vi "Finish_LDA.vi"() -> (1 "LDA Binary output":u16[][](array[numeric])=[[142, 132, 123, 114, 103, 93, 84, 74, 65, 56, 49, 42, 35, 30, 27, 24, 23, 22, 24, 26, 30, 35, 41, 48, 56, 65, 73, 82, 93, 102, 112, 122, 132, 141, 149, 156, 164, 169, 173, 177, 180, 181, 181, 179, 176, 171, 167, 160, 153, 145, 137, 128, 118, 108, 98, 88, 79, 69, 61, 52, 45, 38, 33, 28, 25, 23, 22, 23, 25, 29, 32, 39, 45, 52, 60, 69, 78, 88, 97, 108, 118, 127, 136, 145, 153, 160, 166, 171, 176, 179, 180, 181, 180, 178, 174, 169, 164, 157, 149, 141]], 4 "Repeat Block":bool)   [LabVIEW 2010]
doc: "The Getting Started Analog Input VI illustrates the basic concepts involved in acquiring analog input data from any data acquisition hardware.\n\nThis VI is explained in detail in the Getting Started with Analog Input section of chapter 1 of the Data Acquisition VI Reference Manual. If you are using SCXI, you should read the Getting Started with SCXI section of chapter 1 first.\n\nAfter you have installed and configured your data acquisition hardware as described in the Installation and Configuration section of chapter 1, you can run this VI to verify your hardware configuration. \n\nYou can pop-up on any front panel object for a description.\n\nIf you are using AMUX-64T boards or SCXI hardware, look at the channels control description for instructions on how to address those external channels; otherwise, you can run the VI with default inputs.\n\nOpen the diagram window to see the data acquisition VI usage."
uses:
  Globals/LDA_meas_global_1.vi
  Globals/Meas_global.vi
  Globals/LDA_meas_global_2.vi
panel:
  out "error out":errorcluster
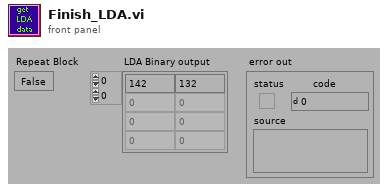
[diagram p1: front panel]
types:
  T1 = typedef "BSA_info_Cluster.ctl" = cluster{"GPIB Address":string, "No of Check Bytes":i32, "Extra Info":string, "COLOUR":u32, "Wavelength (nm)":dbl}
  T2 = cluster{"Burst criterion":enum16{"Envelope", "Pedestal", "Env and ped"}, "Oversize reject level":enum16{"1 (disabled)", "2", "3", "4", "5", "6", "7", "8", "9"}, "Pedestal attenuation":enum16{"0", "6", "12", "18"}, "Record length":enum16{"8", "16", "32", "64"}, "Quality factor":i16}
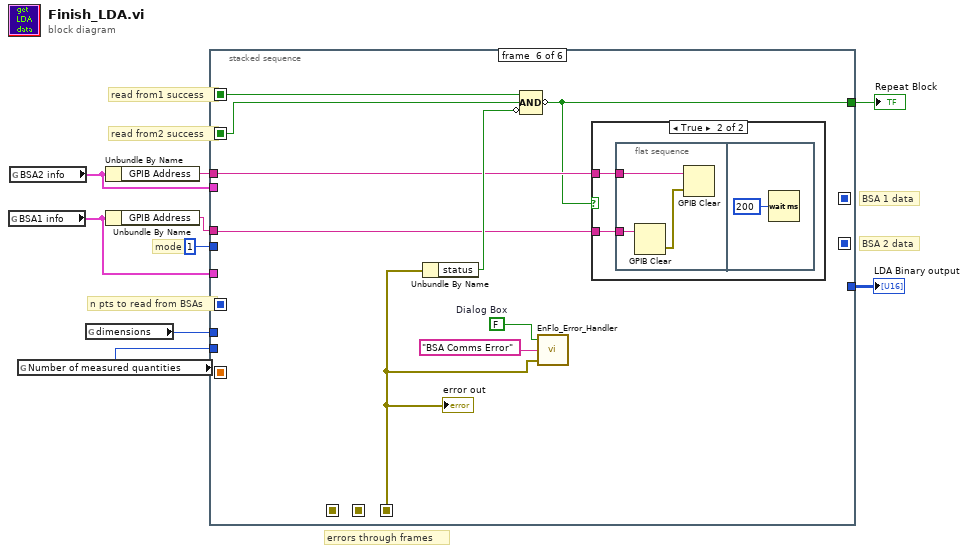
[diagram p0: block diagram]
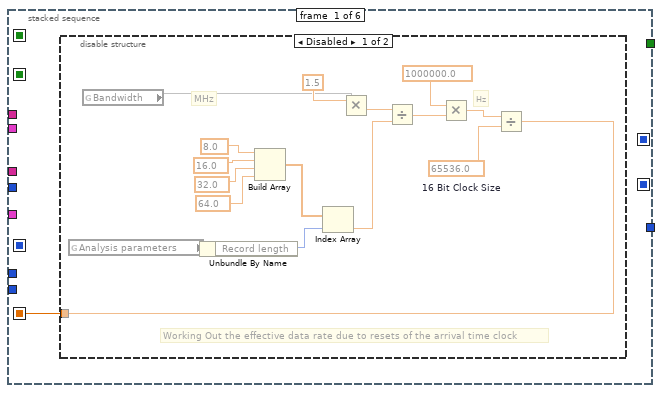
[diagram p2: hidden frame]
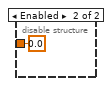
[diagram p3: hidden frame]
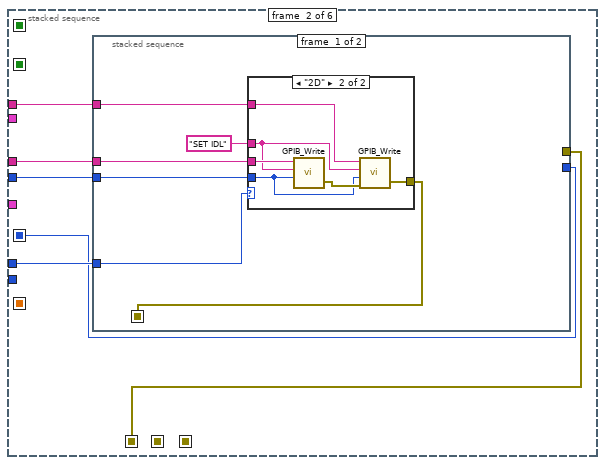
[diagram p4: hidden frame]
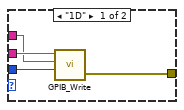
[diagram p5: hidden frame]
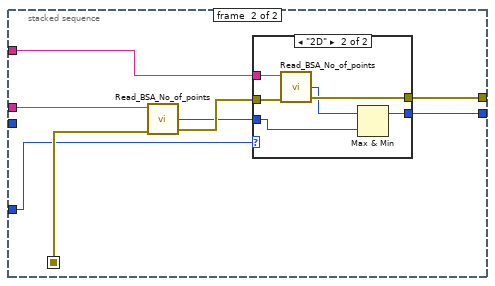
[diagram p6: hidden frame]
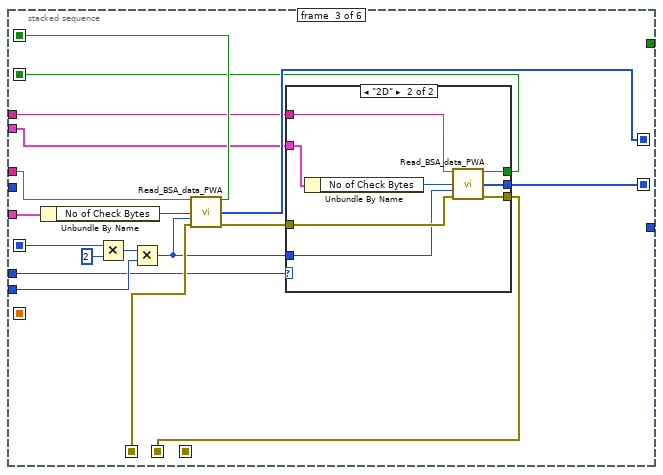
[diagram p8: hidden frame]
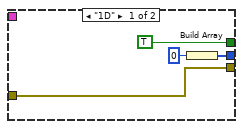
[diagram p9: hidden frame]
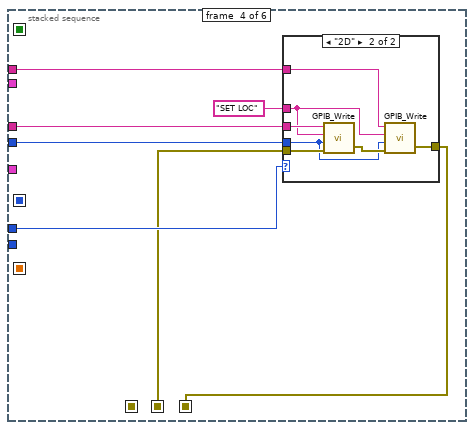
[diagram p10: hidden frame]
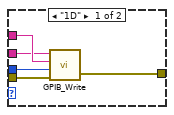
[diagram p11: hidden frame]
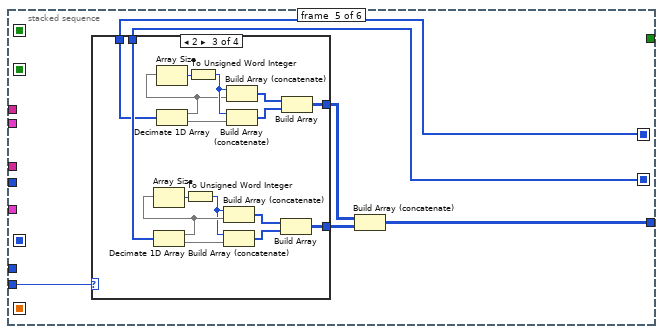
[diagram p12: hidden frame]
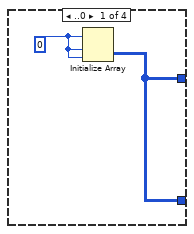
[diagram p13: hidden frame]
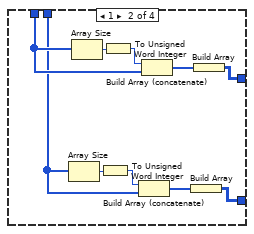
[diagram p14: hidden frame]
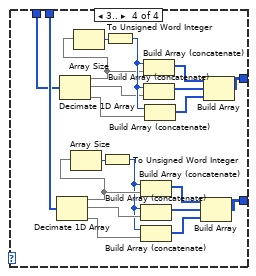
[diagram p15: hidden frame]
diagram:
  # "errors through frames"
  # "BSA 2 data"
  # "BSA 1 data"
  # "read from2 success"
  # "read from1 success"
  # "mode"
  # "n pts to read from BSAs"
  n1 = global read "LDA_meas_global_1.vi" "BSA1 info"() -> (w1:T1)
  n2 = global read "LDA_meas_global_2.vi" "BSA2 info"() -> (w2:T1)
  n3 = global read "LDA_meas_global_1.vi" "Number of measured quantities"() -> (w8:i32)
  n4 = global read "Meas_global.vi" "dimensions"() -> (w6:enum16{"1D", "2D"})
  n5 = Unbundle By Name(w2) -> ("GPIB Address"=w3:string)
  n6 = Unbundle By Name(w1) -> ("GPIB Address"=w7:string)
  n7 = stacked-sequence {
    seq-local: [_ _ w78 _ _ _] -> [_ _ _ _ w119 _]
    seq-local: [_ _ w70 _ _ _] -> [_ _ _ _ w118 _]
    seq-local: [_ _ w82 _ _ _] -> [_ _ _ _ _ w177]
    seq-local: [_ _ w73 _ _ _] -> [_ _ _ _ _ w176]
    seq-local: [_ w28 _ _ _ _] -> [_ _ w75 _ _ _]
    seq-local: [_ _ _ w96 _ _] -> [_ _ _ _ _ w172]
    seq-local: [_ w29 _ _ _ _] -> [_ _ w77 _ _ _]
    seq-local: [w10 _ _ _ _ _] -> [_ _ _ _ _ _]
    seq-local: [_ _ w67 _ _ _] -> [_ _ _ w97 _ _]
    tunnel: w8 -> [_ _ w83 _ w120 _]
    tunnel: i16 1 -> [_ w32 _ w102 _ _]
    tunnel: w7 -> [_ w33 w76 w100 _ w171]
    tunnel: w6 -> [_ w31 w66 w99 _ _]
    tunnel: [_ _ _ _ w115 _] -> w5
    tunnel: [_ _ _ _ _ w169] -> w4
    tunnel: w3 -> [_ w30 w72 w98 _ w170]
    tunnel: w1 -> [_ _ w74 _ _ _]
    tunnel: w2 -> [_ _ w71 _ _ _]
    frame #0 {
      n8 = disable-structure shown="Disabled" {
        disable-tunnel: [w11 0.0] -> w10
        frame Disabled {
          w20 = 65536.0  # 16 Bit Clock Size
          # "Hz"
          # "MHz"
          # "Working Out the effective data rate due to resets of the arrival time clock"
          n9 = global read "LDA_meas_global_1.vi" "Analysis parameters"() -> (w19:T2)
          n10 = global read "LDA_meas_global_1.vi" "Bandwidth"() -> (w25)
          n11 = Unbundle By Name(w19) -> ("Record length"=w13:enum16{"8", "16", "32", "64"})
          n12 = Build Array(8.0, 16.0, 32.0, 64.0) -> (w14:dbl[])
          n13 = Index Array(array=w14, index=w13) -> (element=w12:dbl)
          n14 = Multiply(x=1.5, y=w25) -> (x*y=w24:dbl)
          n15 = Divide(x=w24, y=w12) -> (x/y=w23:dbl)
          n16 = Multiply(x=1000000.0, y=w23) -> (x*y=w21:dbl)
          n17 = Divide(x=w21, y=w20) -> (x/y=w11:dbl)
        }
        frame Enabled {
        }
      }
    }
    frame #1 {
      n18 = stacked-sequence {
        seq-local: [w37 _] -> [_ w56]
        tunnel: w33 -> [w39 w57]
        tunnel: w32 -> [w38 _]
        tunnel: w31 -> [w36 w51]
        tunnel: w30 -> [w34 w55]
        tunnel: [_ w52] -> w29
        tunnel: [_ w50] -> w28
        frame #0 {
          n19 = case shown="\"2D\"" w36 {
            tunnel: w39 -> [w43 w49]
            tunnel: w38 -> [w42 w44]
            tunnel: [w41 w47] -> w37
            tunnel: "SET IDL" -> [w40 w45]
            tunnel: w34 -> [_ w46]
            frame "1D" {
              n20 = call "GPIB_Write.vi"("address string"=w43, "data In"=w40, "mode (0)"=w42) -> ("error out"=w41:errorcluster)  [unwired: 2 in, 1 out]
            }
            frame "2D" {
              n21 = call "GPIB_Write.vi"("address string"=w49, "data In"=w45, "mode (0)"=w44) -> ("error out"=w48:errorcluster)  [unwired: 2 in, 1 out]
              n22 = call "GPIB_Write.vi"("address string"=w46, "data In"=w45, "mode (0)"=w44, "error in"=w48) -> ("error out"=w47:errorcluster)  [unwired: 1 in, 1 out]
            }
          }
        }
        frame #1 {
          n23 = call "Read_BSA_No_of_points.vi"("error in (no error)"=w56, "GPIB Address"=w57) -> ("error out"=w54:errorcluster, "No of samples"=w53:i32)  [unwired: 3 out]
          n24 = case shown="\"2D\"" w51 {
            tunnel: w54 -> [w59 w65]
            tunnel: w55 -> [_ w64]
            tunnel: [w59 w63] -> w50
            tunnel: w53 -> [w58 w61]
            tunnel: [w58 w60] -> w52
            frame "1D" {
            }
            frame "2D" {
              n25 = call "Read_BSA_No_of_points.vi"("error in (no error)"=w65, "GPIB Address"=w64) -> ("error out"=w63:errorcluster, "No of samples"=w62:i32)  [unwired: 3 out]
              n26 = Max & Min(x=w62, y=w61) -> (max(x,y)=w60:i32)  [unwired: 1 out]
            }
          }
        }
      }
    }
    frame #2 {
      n27 = Unbundle By Name(w74) -> ("No of Check Bytes"=w79:i32)
      n28 = Multiply(x=w77, y=2) -> (x*y=w80:i32)
      n29 = Multiply(x=w80, y=w83) -> (x*y=w68:i32)
      n30 = call "Read_BSA_data_PWA.vi"("GPIB Address"=w76, "No of Check Bytes"=w79, "Bytes per block"=w68, "error in (no error)"=w75) -> ("transmission okay"=w82:bool, "array of velocity data"=w78:u16[], "error out"=w69:errorcluster)  [unwired: 9 out]
      n31 = case shown="\"2D\"" w66 {
        tunnel: [w86 w95] -> w70
        tunnel: [TRUE ("transmission okay") w93] -> w73
        tunnel: [w84 w89] -> w67
        tunnel: w71 -> [_ w92]
        tunnel: w72 -> [_ w91]
        tunnel: w69 -> [w84 w90]
        tunnel: w68 -> [_ w88]
        frame "1D" {
          n32 = Build Array(u16 0) -> (w86:u16[])
        }
        frame "2D" {
          n33 = Unbundle By Name(w92) -> ("No of Check Bytes"=w94:i32)
          n34 = call "Read_BSA_data_PWA.vi"("GPIB Address"=w91, "No of Check Bytes"=w94, "Bytes per block"=w88, "error in (no error)"=w90) -> ("transmission okay"=w93:bool, "array of velocity data"=w95:u16[], "error out"=w89:errorcluster)  [unwired: 9 out]
        }
      }
    }
    frame #3 {
      n35 = case shown="\"2D\"" w99 {
        tunnel: w102 -> [w107 w110]
        tunnel: "SET LOC" -> [w106 w109]
        tunnel: w100 -> [w105 w114]
        tunnel: w97 -> [w104 w113]
        tunnel: [w103 w111] -> w96
        tunnel: w98 -> [_ w108]
        frame "1D" {
          n36 = call "GPIB_Write.vi"("address string"=w105, "data In"=w106, "mode (0)"=w107, "error in"=w104) -> ("error out"=w103:errorcluster)  [unwired: 1 in, 1 out]
        }
        frame "2D" {
          n37 = call "GPIB_Write.vi"("address string"=w114, "data In"=w109, "mode (0)"=w110, "error in"=w113) -> ("error out"=w112:errorcluster)  [unwired: 1 in, 1 out]
          n38 = call "GPIB_Write.vi"("address string"=w108, "data In"=w109, "mode (0)"=w110, "error in"=w112) -> ("error out"=w111:errorcluster)  [unwired: 1 in, 1 out]
        }
      }
    }
    frame #4 {
      n39 = case shown="2" w120 {
        tunnel: w119 -> [_ w124 w133 w149]
        tunnel: w118 -> [_ w123 w148 w168]
        tunnel: [w121 w132 w147 w167] -> w117
        tunnel: [w121 w131 w146 w166] -> w116
        frame ..0 {
          w122 = u16 0
          n40 = Initialize Array(w122, w122, w122) -> (w121:u16[][])
        }
        frame 1 {
          n41 = Array Size(array=w123) -> (size(s)=w130:i32)
          n42 = Array Size(array=w124) -> (size(s)=w125:i32)
          n43 = To Unsigned Word Integer(number=w130) -> (unsigned 16bit integer=w129:u16)
          n44 = To Unsigned Word Integer(number=w125) -> (unsigned 16bit integer=w126:u16)
          n45 = Build Array (concatenate)(w129, w123) -> (w128:u16[])
          n46 = Build Array (concatenate)(w126, w124) -> (w127:u16[])
          n47 = Build Array(w128) -> (w131:u16[][])
          n48 = Build Array(w127) -> (w132:u16[][])
        }
        frame 2 {
          n49 = Decimate 1D Array(w148) -> (w145:u16[], w143:u16[])
          n50 = Array Size(array=w145) -> (size(s)=w144:i32)
          n51 = Decimate 1D Array(w133) -> (w134:u16[], w136:u16[])
          n52 = Array Size(array=w134) -> (size(s)=w135:i32)
          n53 = To Unsigned Word Integer(number=w144) -> (unsigned 16bit integer=w142:u16)
          n54 = To Unsigned Word Integer(number=w135) -> (unsigned 16bit integer=w137:u16)
          n55 = Build Array (concatenate)(w142, w145) -> (w141:u16[])
          n56 = Build Array (concatenate)(w142, w143) -> (w140:u16[])
          n57 = Build Array (concatenate)(w137, w134) -> (w138:u16[])
          n58 = Build Array (concatenate)(w137, w136) -> (w139:u16[])
          n59 = Build Array(w141, w140) -> (w146:u16[][])
          n60 = Build Array(w138, w139) -> (w147:u16[][])
        }
        frame 3.. {
          n61 = Decimate 1D Array(w168) -> (w165:u16[], w163:u16[], w162:u16[])
          n62 = Decimate 1D Array(w149) -> (w150:u16[], w152:u16[], w153:u16[])
          n63 = Array Size(array=w165) -> (size(s)=w164:i32)
          n64 = Array Size(array=w150) -> (size(s)=w151:i32)
          n65 = To Unsigned Word Integer(number=w164) -> (unsigned 16bit integer=w161:u16)
          n66 = To Unsigned Word Integer(number=w151) -> (unsigned 16bit integer=w154:u16)
          n67 = Build Array (concatenate)(w161, w165) -> (w160:u16[])
          n68 = Build Array (concatenate)(w161, w163) -> (w159:u16[])
          n69 = Build Array (concatenate)(w161, w162) -> (w158:u16[])
          n70 = Build Array (concatenate)(w154, w150) -> (w155:u16[])
          n71 = Build Array (concatenate)(w154, w152) -> (w156:u16[])
          n72 = Build Array (concatenate)(w154, w153) -> (w157:u16[])
          n73 = Build Array(w160, w159, w158) -> (w166:u16[][])
          n74 = Build Array(w155, w156, w157) -> (w167:u16[][])
        }
      }
      n75 = Build Array (concatenate)(w117, w116) -> (w115:u16[][])
    }
    frame #5 {
      w175 = FALSE  # Dialog Box
      n76 = Unbundle By Name(w172) -> ("status"=w173:bool)
      n77 = Compound Arithmetic op=AND(w177, w176, invert w173) -> (invert w169:bool)
      n78 = call "EnFlo_Error_Handler.vi"("error in (no error)"=w172, "Error Type"="BSA Comms Error", "Dialog Box (T)"=w175) -> ()  [unwired: 3 out]
      n79 = case shown="True" w169 {
        tunnel: w171 -> [_ w179]
        tunnel: w170 -> [_ w178]
        frame False {
        }
        frame True {
          n80 = flat-sequence {
            tunnel: w179 -> [w182]
            tunnel: w178 -> [w181]
            frame #0 {
              n81 = GPIB Clear(3:w182) -> (0:w180:errorcluster)  [unwired: 1 in, 1 out]
              n82 = GPIB Clear(2:w180, 3:w181) -> ()  [unwired: 2 out]
            }
            frame #1 {
              n83 = Wait (ms)(milliseconds to wait=u32 200) -> ()  [unwired: 1 out]
            }
          }
        }
      }
      "error out" <- w172
    }
  }
  "LDA Binary output" <- w5
  "Repeat Block" <- w4
